vi "2-1.vi"() -> ()   [LabVIEW 2022 SP3]
panel:
  out "耗费时间（s）":dbl
  out "随机数个数":dbl
  out "产生的随机整数":dbl
  in  "指定的数":dbl
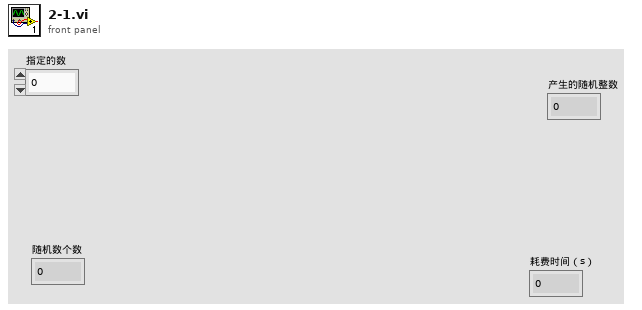
[diagram p1: front panel]
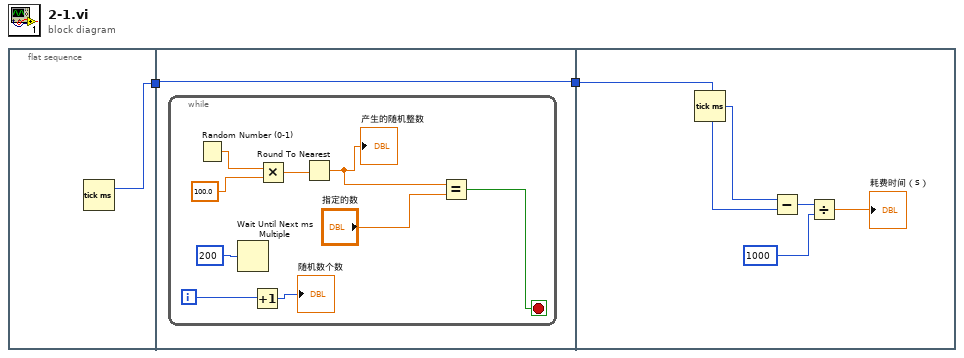
[diagram p0: block diagram]
diagram:
  n1 = flat-sequence {
    tunnel: [w3] -> w2
    tunnel: w2 -> [w4]
    tunnel: [w4] -> w1
    tunnel: w1 -> [w17]
    frame #0 {
      n2 = Tick Count (ms)() -> (millisecond timer value=w3:u32)
    }
    frame #1 {
      n3 = while {
        i -> [w10]
        stop <- w7 stop-if-true
        n4 = Random Number (0-1)() -> (number: 0 to 1=w13:dbl)
        n5 = Wait Until Next ms Multiple(millisecond multiple=200) -> ()  [unwired: 1 out]
        n6 = Increment(x=w10) -> (x+1=→"随机数个数":i32)
        n7 = Multiply(x=w13, y=100.0) -> (x*y=w6:dbl)
        n8 = Round To Nearest(number=w6) -> (nearest integer value=w5:dbl)
        "产生的随机整数" <- w5
        n9 = Equal?(x=w5, y="指定的数") -> (x = y?=w7:bool)
      }
    }
    frame #2 {
      n10 = Tick Count (ms)() -> (millisecond timer value=w18:u32)
      n11 = Subtract(x=w18, y=w17) -> (x-y=w15:u32)
      n12 = Divide(x=w15, y=1000) -> (x/y=→"耗费时间（s）":dbl)
    }
  }
